vi "Peak Detection and Display (Renan).vi"() -> ()   [LabVIEW 2020]
doc: "Demonstrates the use of the Peak Detector VI."
uses:
  <vilib>/Analysis/3filter.llb/Elliptic Filter (DBL).vi
  <vilib>/Analysis/NI_AALBase.lvlib
  <vilib>/Analysis/NI_AAL_SigProc.lvlib
panel:
  in  "valley detector width":i32=3 min=3
  in  "signal source":u16(ring) items=["Filtered Noise", "Sinc", "Sin + Cos"]
  out "valleys found":i32
  in  "Stop":bool
  in  "filter order":i32=2
  in  "noise seed":i32=1
  in  "peak detector width":i32=3 min=3
  out "Signal Plot":cluster{"Locations":dbl[], "Amplitudes":dbl[]}[](graph)
  out "peaks found":i32
  # "Overview: Demonstrates the use of the Peak Detector VI to find peaks and valleys in a variety of signals.\nRequirements: LabVIEW Full Development System\nInstructions:\n1. Run the VI.\n2. Within the Signal Plot, move the horizontal cursors to adjust the peak detector threshold levels (red for Peaks, blue for Valleys).\n3. Change the signal source along with the noise seed and filter order to modify the signal shape.\n4. Change the peak detector width to observe how smoothing increases with width.\n5. Click Stop to stop the VI."
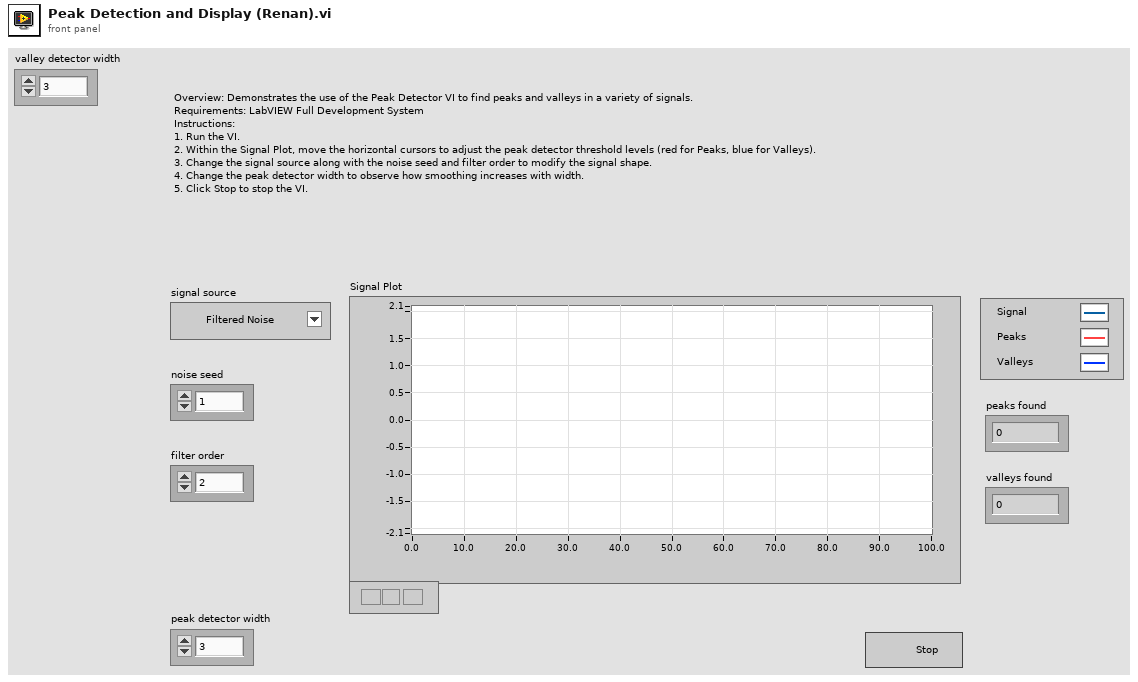
[diagram p1: front panel]
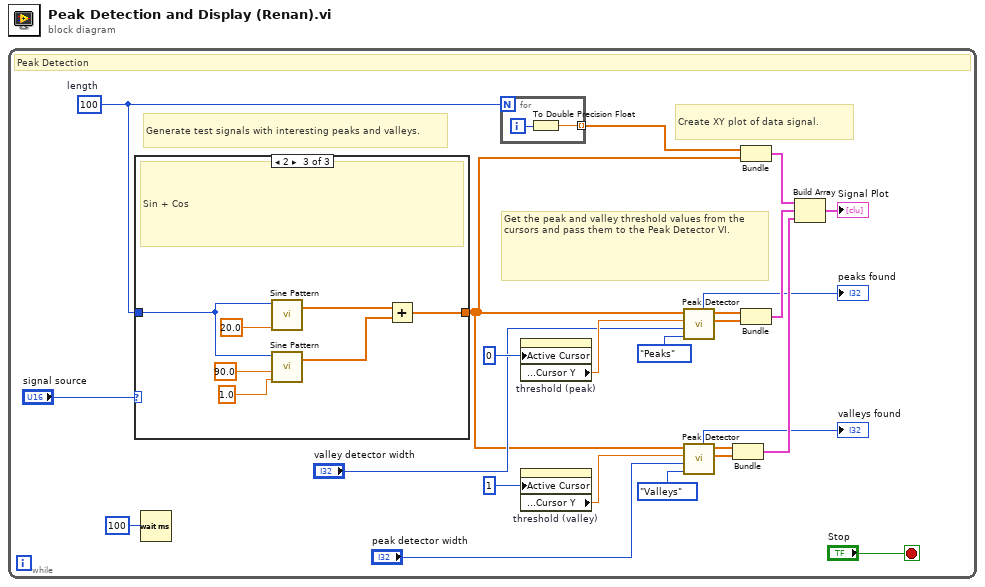
[diagram p0: block diagram]
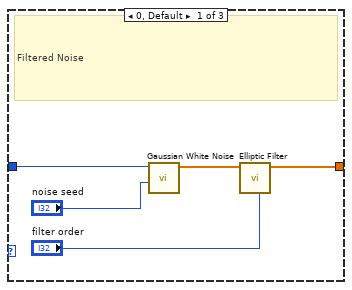
[diagram p2: hidden frame]
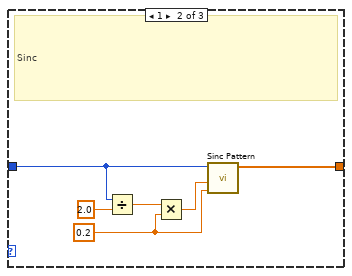
[diagram p3: hidden frame]
diagram:
  n1 = while {
    stop <- "Stop" stop-if-true
    w11 = 100  # length
    # "Get the peak and valley threshold values from the cursors and pass them to the Peak Detector VI."
    # "Create XY plot of data signal."
    # "Generate test signals with interesting peaks and valleys."
    # "Peak Detection"
    n2 = case shown="2" "signal source" {
      tunnel: [w29 w35 w43] -> w1
      tunnel: w11 -> [w31 w34 w41]
      frame 0, Default {
        # "Filtered Noise"
        n3 = call <vilib>:"Gaussian White Noise.vi"("seed"="noise seed", "samples"=w31) -> ("Gaussian noise pattern"=w30:dbl[])  [unwired: 8 in, 1 out]
        n4 = call-poly <vilib>:"Elliptic Filter.vi"("order"="filter order", "X"=w30) -> ("Filtered X"=w29:dbl[])  [unwired: 8 in, 1 out]
      }
      frame 1 {
        w32 = 0.2
        # "Sinc"
        n5 = Divide(x=w34, y=2.0) -> (x/y=w37:dbl)
        n6 = Multiply(x=w37, y=w32) -> (x*y=w36:dbl)
        n7 = call <vilib>:"Sinc Pattern.vi"("delta t"=w32, "delay"=w36, "samples"=w34) -> ("Sinc Pattern"=w35:dbl[])  [unwired: 1 in, 1 out]
      }
      frame 2 {
        # "Sin + Cos"
        n8 = call <vilib>:"Sine Pattern.vi"("cycles"=20.0, "samples"=w41) -> ("Sinusoidal Pattern"=w44:dbl[])  [unwired: 2 in, 1 out]
        n9 = call <vilib>:"Sine Pattern.vi"("cycles"=1.0, "phase(degrees)"=90.0, "samples"=w41) -> ("Sinusoidal Pattern"=w42:dbl[])  [unwired: 1 in, 1 out]
        n10 = Add(x=w44, y=w42) -> (x+y=w43:dbl[])
      }
    }
    n11 = Wait (ms)(milliseconds to wait=u32 100) -> ()  [unwired: 1 out]
    n12 = for {
      N: w11 -> [_]
      tunnel: [w25] -> w12 mode=indexing
      i -> [w26]
      n13 = To Double Precision Float(number=w26) -> (double precision float=w25:dbl)
    }
    n14 = property on="threshold (peak)" class="XYGraph (strict)"("Active Cursor"=u32 0) -> ("Cursor.Cursor Position:Cursor Y"=w4:dbl)  [unwired: 2 in, 2 out]
    n15 = property on="threshold (valley)" class="XYGraph (strict)"("Active Cursor"=u32 1) -> ("Cursor.Cursor Position:Cursor Y"=w5:dbl)  [unwired: 2 in, 2 out]
    n16 = call <vilib>:"Peak Detector.vi"("peaks/valleys"=enum32{"Peaks", "Valleys"}."Peaks", "width"="valley detector width", "threshold"=w4, "X"=w1) -> ("Amplitudes"=w22:dbl[], "Locations"=w14:dbl[], "# found"=→"peaks found":i32)  [unwired: 3 in, 2 out]
    n17 = call <vilib>:"Peak Detector.vi"("peaks/valleys"=enum32{"Peaks", "Valleys"}."Valleys", "width"="peak detector width", "threshold"=w5, "X"=w1) -> ("Amplitudes"=w19:dbl[], "Locations"=w20:dbl[], "# found"=→"valleys found":i32)  [unwired: 3 in, 2 out]
    n18 = Bundle("Locations"=w20, "Amplitudes"=w19) -> (w17:cluster{"Locations":dbl[], "Amplitudes":dbl[]})  [unwired: 1 in]
    n19 = Bundle(w12, "Sinc Pattern"=w1) -> (w24:cluster{dbl[], "Sinc Pattern":dbl[]})  [unwired: 1 in]
    n20 = Bundle("Locations"=w14, "Amplitudes"=w22) -> (w21:cluster{"Locations":dbl[], "Amplitudes":dbl[]})  [unwired: 1 in]
    n21 = Build Array(w24, w21, w17) -> (→"Signal Plot":cluster{"Locations":dbl[], "Amplitudes":dbl[]}[])
  }
